vi "PhaseModulationExample.vi"() -> ()   [LabVIEW 2013]
panel:
  in  "Modulation Frequency (10000)":dbl=10000.0
  in  "Peak Deviation (90)":dbl=90.0
  in  "Modulation Waveform":i32(ring) items=["Arbitrary User1"=200, "Arbitrary User2"=201, "Arbitrary User3"=202, "Arbitrary User4"=203, "Edit Memory"=204, "Sine"=1, "Square"=2, "Noise"=100, "Ramp down"=5, "Ramp up"=4, "Triangle"=3]
  in  "Enabled":bool
  in  "Source (0: Internal)":i32(ring) items=["Internal", "External"]
  in  "channel name (\"1\")":string
  in  "resource name":refnum<k15>
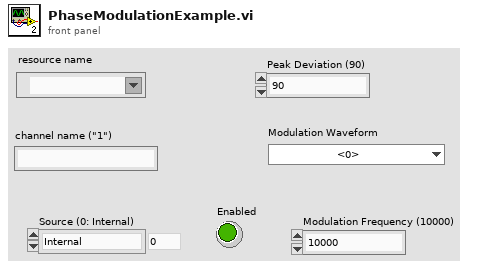
[diagram p1: front panel]
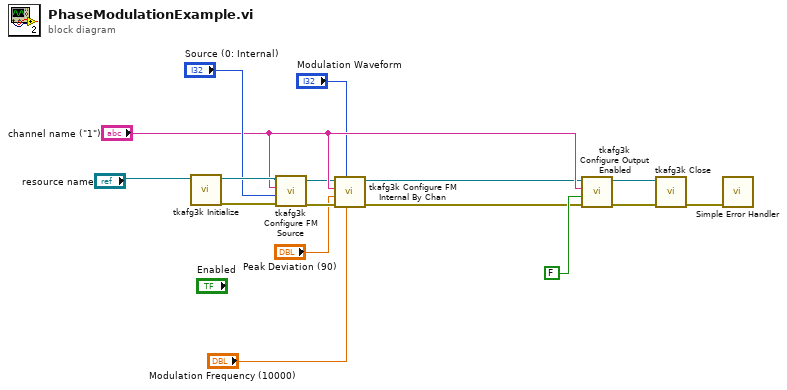
[diagram p0: block diagram]
diagram:
  n1 = call <instrlib>:"tkafg3k Initialize.vi"("resource name"="resource name") -> ("error out"=w10:errorcluster, "instrument handle out"=w11:refnum<k15>)  [unwired: 9 in]
  n2 = call <instrlib>:"tkafg3k Configure FM Source.vi"("error in (no error)"=w10, "source (0: Internal)"="Source (0: Internal)", "channel name (\"1\")"="channel name (\"1\")", "instrument handle"=w11) -> ("error out"=w6:errorcluster, "instrument handle out"=w7:refnum<k15>)  [unwired: 6 in]
  n3 = call <instrlib>:"tkafg3k Configure FM Internal By Chan.vi"("Modulation Frequency (10000)"="Modulation Frequency (10000)", "Modulation Waveform (1: Sine)"="Modulation Waveform", "error in (no error)"=w6, "Peak Deviation (1000000)"="Peak Deviation (90)", "Channel Name (\"1\")"="channel name (\"1\")", "instrument handle"=w7) -> ("error out"=w3:errorcluster, "instrument handle out"=w4:refnum<k15>)  [unwired: 4 in]
  n4 = call <instrlib>:"tkafg3k Configure Output Enabled.vi"("error in (no error)"=w3, "channel enabled (True)"=FALSE, "channel name (\"1\")"="channel name (\"1\")", "instrument handle"=w4) -> ("error out"=w13:errorcluster, "instrument handle out"=w14:refnum<k15>)  [unwired: 6 in]
  n5 = call <instrlib>:"tkafg3k Close.vi"("error in (no error)"=w13, "instrument handle"=w14) -> ("error out"=w12:errorcluster)  [unwired: 9 in]
  n6 = call <vilib>:"Simple Error Handler.vi"("error in (no error)"=w12) -> ()  [unwired: 1 in, 8 out]
